vi "raster-scanning.vi"() -> ()   [LabVIEW 2017]
uses:
  controls/boolean_info.ctl
  raster-scan-params.ctl
  controls/PI-params.ctl
  <vilib>/rvi/Emulation/niFpgaGetClockAttributes.vi
  <vilib>/rvi/Emulation/niFpgaSctlEmulationGetInTimedLoop.vi
  <vilib>/rvi/Emulation/niFpgaEmulationReportErrorSimple.vi
  <vilib>/rvi/eio/common/nirviEmuTemplateMethod_errors.vi
  <vilib>/rvi/Emulation/niFpgaEmulationIsFPGAContextNoSignature.vi
  <vilib>/rvi/DataTransferAndStorage/Container/Common/niFpgaContainerGetUniqueNameForEmu.vi
  <vilib>/rvi/Memory/Memory_Emulation/niFpgaMemoryEmulationCacheClearOnFirstRun.vi
  <vilib>/rvi/Memory/Memory_Emulation/nirvimemoryEmulationManagerCache_MakeExclusive.vi
  <vilib>/rvi/Memory/Memory_Emulation/niFpgaMemoryEmulationValidateCache.vi
  <vilib>/rvi/Memory/Memory_Emulation/nirvimemoryEmulationManagerCache_InsertValue.vi
  <vilib>/Utility/error.llb/Clear Errors.vi
  <vilib>/rvi/Memory/Memory_Emulation/nirvimemoryEmulationManagerCache_ReleaseExclusive.vi
  <vilib>/rvi/Memory/Memory_Emulation/nirvimemoryEmulationManagerCache_GetValue.vi
  <vilib>/rvi/Memory/Memory_Emulation/nirvimemoryEmulationManagerCache_SetValue.vi
  <vilib>/rvi/Emulation/niFpgaProcessEmulError.vi
  <vilib>/rvi/DataTransferAndStorage/Container/Common/niFpgaContainerExecOnDevCompGetState.vi
  <vilib>/rvi/Emulation/niFpgaCriticalErrorInLSC.vi
  <vilib>/eio/EIONode/EIONode.xnode
  <vilib>/rvi/DataTransferAndStorage/Container/XNode/niFpgaContainer.xnode
  <vilib>/rvi/DataTransferAndStorage/Register/Emulation/niFpgaRegisterEmulation.vi
  <vilib>/rvi/DataTransferAndStorage/Register/Emulation/niFpgaRegisterEmulationRefIn.vi
  libimaging-cs.lvlib
  FPGA-data-logging.lvlib
panel:
  in  "ze_sched_thresh":sgl
  in  "KI_derate":sgl
  in  "raster-scan-params":T1={"TsTicks"=1600, "Stop"=TRUE, "TOL"=0.3, "ramp-rate"=0.0, "z-u-max"=5.0, "PI-params"={"Ki"=0.001, "setpoint"=0.0}, "Num"=[-0.00254, 0.000408, 0.00295, 0.0, 0.0, 0.0, 0.0, 0.0, 0.0], "TF Order"=2, "Den"=[0.982758, -1.98194, 1.0, 0.0, 0.0, 0.0, 0.0, 0.0, 0.0]} {"z-u-max" format="%#_13g"; "TOL" format="%#_13g"}
  in  "Z-settle-N":i16
  in  "do_xy_CL":bool
  in  "do-Dz":bool
  out "boolean errors":T3
  in  "xy-init":fxp<+/-,16,5>[](array[numeric])=[0.0, 0.0]
  in  "Ki-xy":sgl=0.001 format="%#_13g"
  in  "xy-bound":sgl
  in  "trigger-0":bool
  in  "u(0)":sgl format="%#_13g"
  out "e(0) (threshhold init)":fxp<+/-,16,5>
  out "current-case":i16
  out "DAC-zaxis":sgl
  out "ADC-zaxis":fxp<+/-,24,5>
  in  "raise-constant":sgl
  # "DIAGNOSTICS"
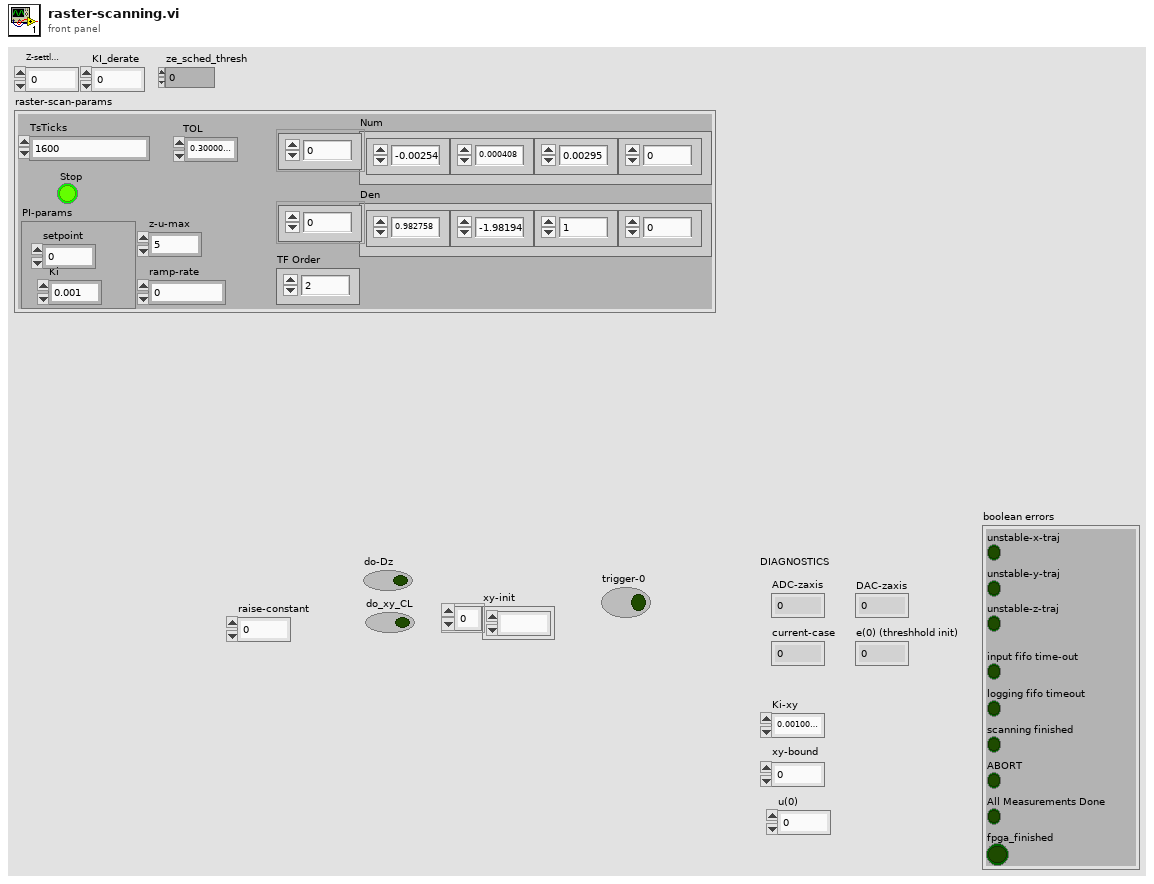
[diagram p1: front panel]
types:
  T1 = typedef "raster-scan-params.ctl" = cluster{"TsTicks":u32, "Stop":bool, "TOL":sgl, "ramp-rate":sgl, "z-u-max":sgl, "PI-params":T2, "Num":sgl[], "TF Order":i32, "Den":sgl[]}
  T2 = typedef "PI-params.ctl" = cluster{"Ki":sgl, "setpoint":sgl}
  T3 = typedef "boolean_info.ctl" = cluster{"unstable-z-traj":bool, "input fifo time-out":bool, "logging fifo timeout":bool, "scanning finished":bool, "unstable-x-traj":bool, "unstable-y-traj":bool, "ABORT":bool, "All Measurements Done":bool, "fpga_finished":bool}
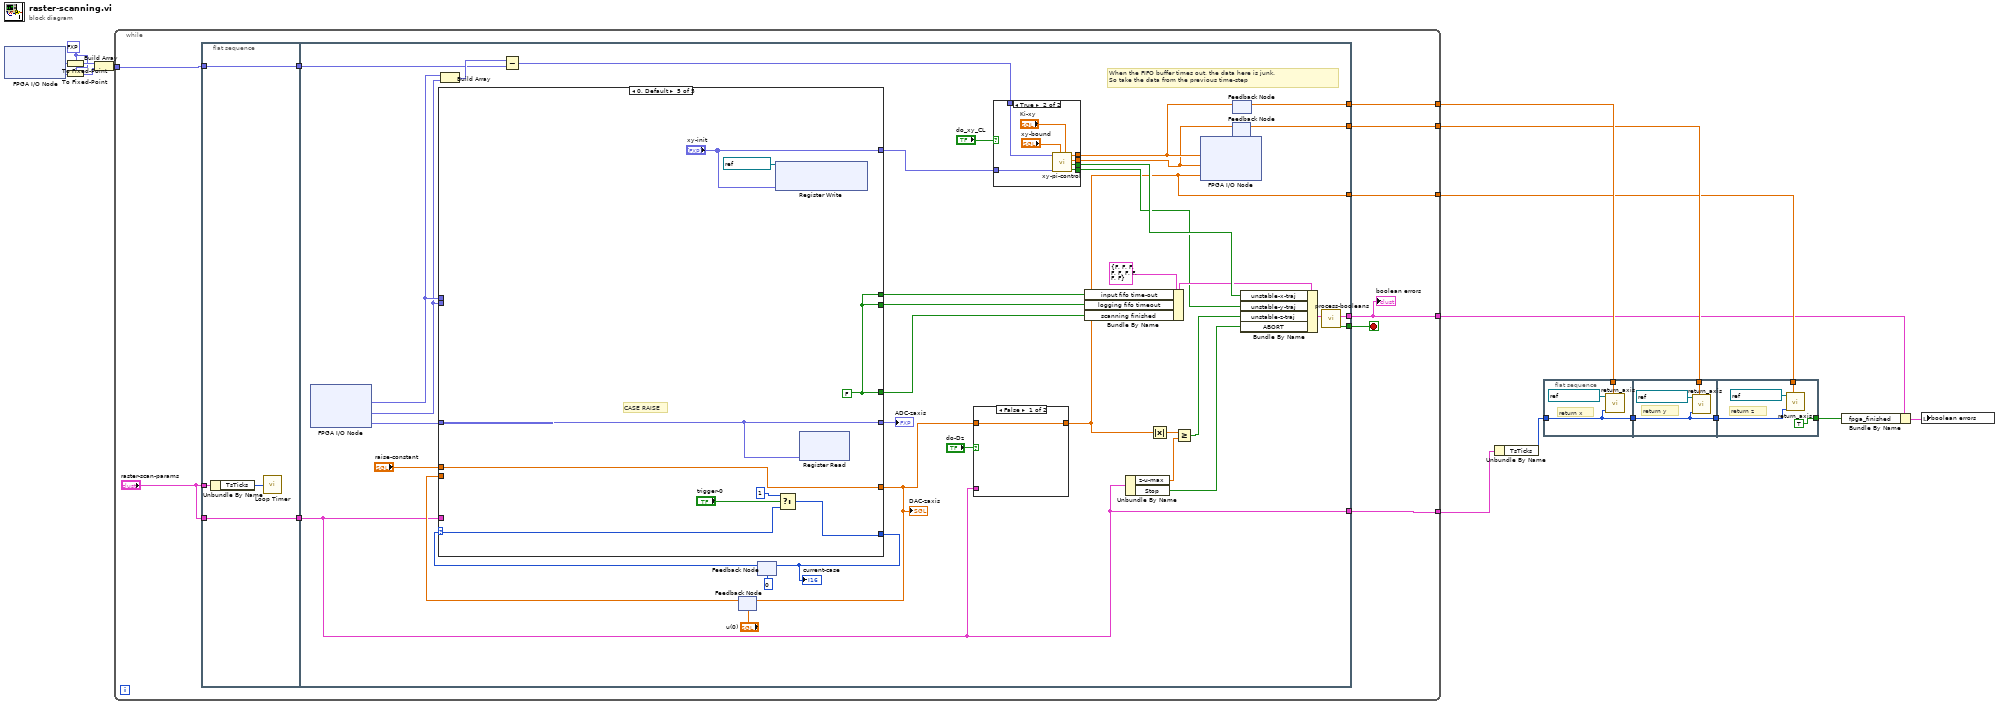
[diagram p0: block diagram]
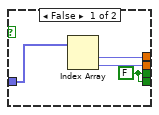
[diagram p2: hidden frame]
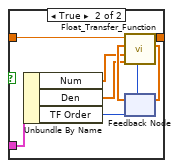
[diagram p3: hidden frame]
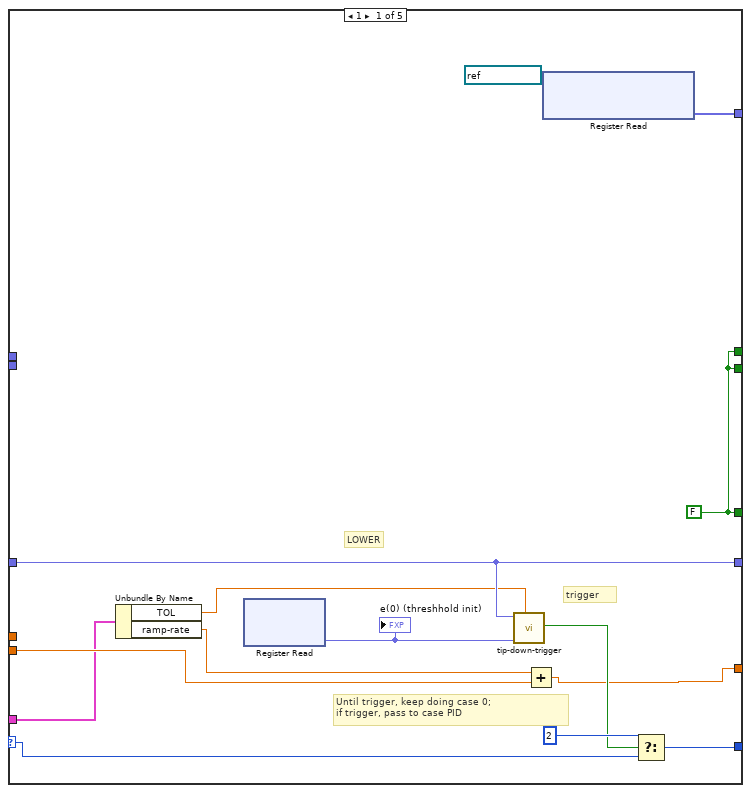
[diagram p4: hidden frame]
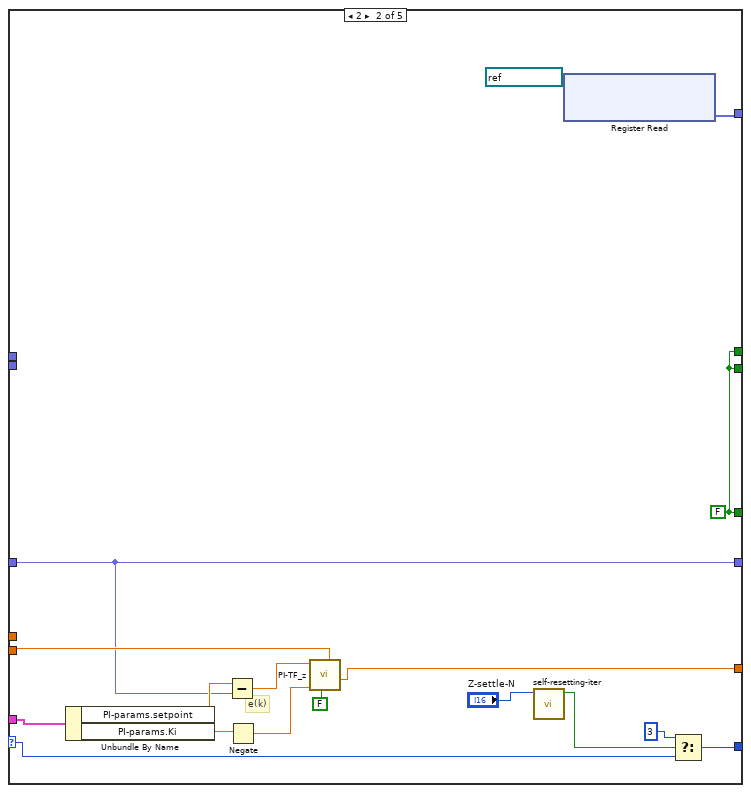
[diagram p5: hidden frame]
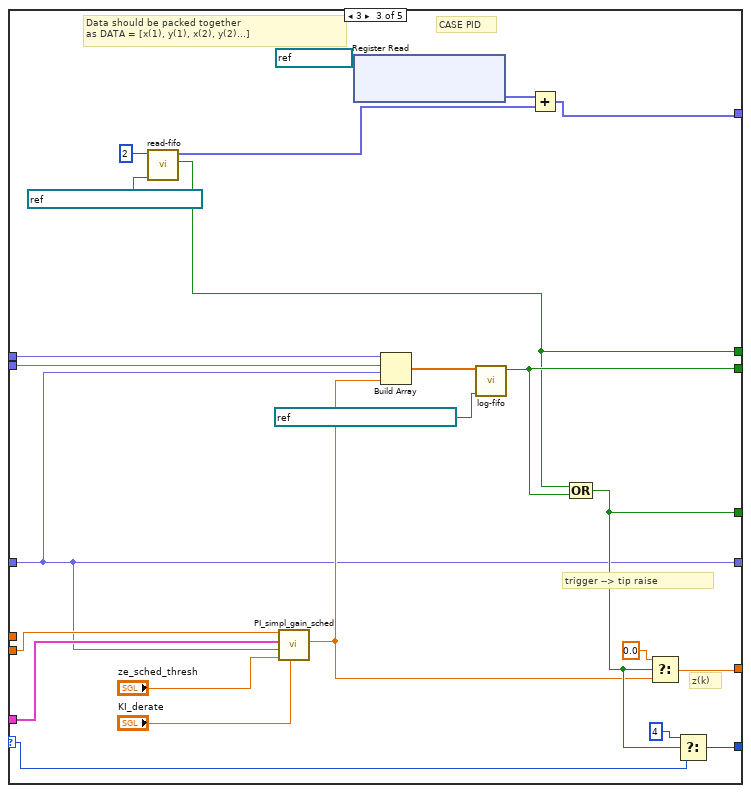
[diagram p6: hidden frame]
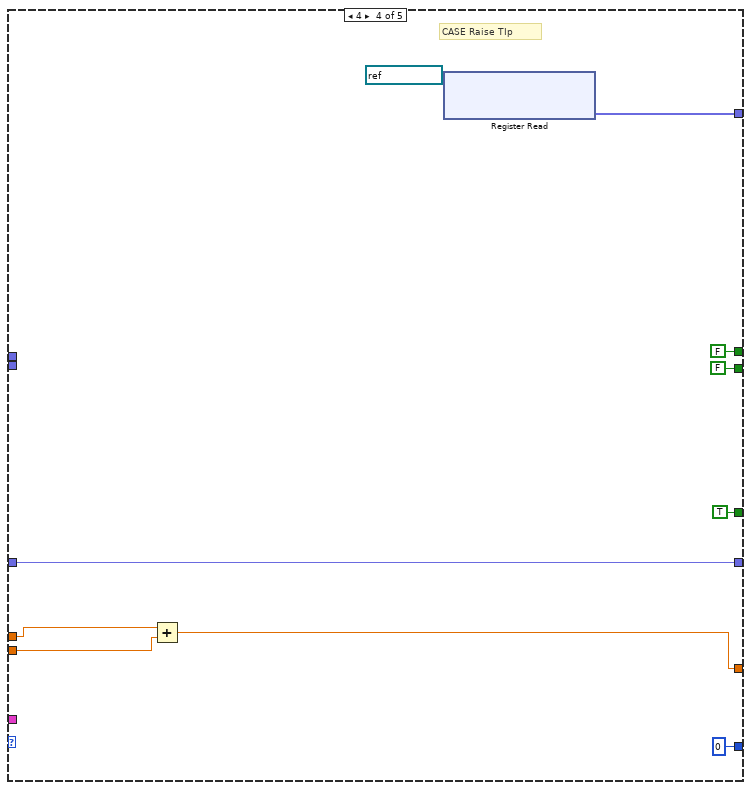
[diagram p7: hidden frame]
diagram:
  w2 = fxp<+/-,16,5> 0.0 ("fixed-point type")
  n1 = xnode "FPGA I/O Node"() -> ("Mod2/AI0"=w5:fxp<+/-,24,5>, "Mod2/AI1"=w3:fxp<+/-,24,5>)  [unwired: 2 in, 2 out]
  n2 = To Fixed-Point(fixed-point type=w2, number=w5) -> (fixed-point=w6:fxp<+/-,16,5>)
  n3 = To Fixed-Point(fixed-point type=w2, number=w3) -> (fixed-point=w4:fxp<+/-,16,5>)
  n4 = Build Array(w6, w4) -> (w1:fxp<+/-,16,5>[])
  n5 = while {
    tunnel: [w25] -> w16
    tunnel: [w24] -> w14
    tunnel: [w21] -> w8
    tunnel: [w23] -> w12
    tunnel: [w22] -> w13
    tunnel: w1 -> [w19]
    stop <- w18 stop-if-true
    n6 = flat-sequence {
      tunnel: "raster-scan-params" -> [w29]
      tunnel: [w28] -> w26
      tunnel: "raster-scan-params" -> [w28]
      tunnel: w19 -> [w27]
      tunnel: [w27] -> w20
      tunnel: w26 -> [w37]
      tunnel: [w59] -> w24
      tunnel: [w37] -> w25
      tunnel: [w33] -> w21
      tunnel: [w39] -> w23
      tunnel: [w52] -> w22
      tunnel: w20 -> [w46]
      tunnel: [w31] -> w18
      frame #0 {
        n7 = Unbundle By Name(w29) -> ("TsTicks"=w30:u32)
        n8 = call "Loop Timer"("Count(Ticks)"=w30) -> ()  [unwired: 1 out]
      }
      frame #1 {
        # "When the FIFO buffer times out, the data here is junk.\nSo take the data from the previous time-step"
        n9 = xnode "FPGA I/O Node"() -> ("Mod2/AI0"=w56:fxp<+/-,24,5>, "Mod2/AI1"=w55:fxp<+/-,24,5>, "Mod2/AI2"=w67:fxp<+/-,24,5>)  [unwired: 3 in, 3 out]
        n10 = Build Array(w56, w55) -> (w47:fxp<+/-,24,5>[])
        n11 = Subtract(x=w47, y=w46) -> (x-y=w45:fxp<+/-,25,6>[])
        n12 = feedback #1("u(0)") -> (w62:sgl)
        n13 = feedback #2(i16 0 ("f")) -> (w63:i16)
        n14 = case shown="0, Default" w63 {
          selector: w63 -> [w91 w108 w136 _ w157]
          tunnel: w62 -> [w102 w113 w124 w152 _]
          tunnel: w67 -> [w99 w106 w122 w146 w162]
          tunnel: [w99 w106 w122 w146 w162] -> w66
          tunnel: [w101 w110 w142 i16 0 ("f") w160] -> w64
          tunnel: w55 -> [_ _ w140 _ _]
          tunnel: w56 -> [_ _ w139 _ _]
          tunnel: [w92 w105 w137 TRUE ("Timed Out?") w159] -> w32
          tunnel: [w96 w112 w138 w151 w156] -> w38
          tunnel: w37 -> [w95 w114 w123 _ _]
          tunnel: [w92 w105 w130 FALSE ("Timed Out?") w159] -> w43
          tunnel: [w92 w105 w134 FALSE ("Timed Out?") w159] -> w44
          tunnel: [w89 w103 w127 w144 "xy-init"] -> w51
          tunnel: "raise-constant" -> [_ _ _ w153 w156]
          frame 1 {
            w92 = FALSE ("Timed Out?")
            # "Until trigger, keep doing case 0;\nif trigger, pass to case PID"
            # "LOWER"
            # "trigger"
            n15 = Unbundle By Name(w95) -> ("TOL"=w94:sgl, "ramp-rate"=w93:sgl)
            n16 = xnode ("Register Read")() -> ("Data"=w97:fxp<+/-,16,5>)  [unwired: 1 in, 1 out]
            "e(0) (threshhold init)" <- w97
            n17 = call "tip-down-trigger.vi"("TOL"=w94, "Vo"=w97, "e(k)"=w99) -> ("trigger"=w98:bool)  [unwired: 8 in]
            n18 = Add(x=w93, y=w102) -> (x+y=w96:sgl)
            n19 = xnode ("Register Read")("Register In"=refnum<k21> "xy_init") -> ("Data"=w89:fxp<+/-,17,6>[])  [unwired: 1 out]
            n20 = Select(t=i16 2, s=w98, f=w91) -> (s? t:f=w101:i16)
          }
          frame 2 {
            w105 = FALSE ("Timed Out?")
            # "e(k)"
            n21 = Unbundle By Name(w114) -> ("PI-params.setpoint"=w119:sgl, "PI-params.Ki"=w116:sgl)
            n22 = Subtract(x=w119, y=w106) -> (x-y=w117:sgl)
            n23 = Negate(x=w116) -> (-x=w115:sgl)
            n24 = call "PI-TF_z.vi"("u(k-1)"=w113, "reset"=FALSE, "Ki"=w115, "e(k)"=w117) -> ("u(k)"=w112:sgl)  [unwired: 7 in]
            n25 = call "self-resetting-iter.vi"("N"="Z-settle-N") -> ("Boolean"=w109:bool)  [unwired: 9 in, 1 out]
            n26 = xnode ("Register Read")("Register In"=refnum<k21> "xy_init") -> ("Data"=w103:fxp<+/-,17,6>[])  [unwired: 1 out]
            n27 = Select(t=i16 3, s=w109, f=w108) -> (s? t:f=w110:i16)
          }
          frame 3 {
            # "Data should be packed together\nas DATA = [x(1), y(1), x(2), y(2)...]"
            # "trigger --> tip raise"
            # "z(k)"
            # "CASE PID"
            n28 = call "read-fifo.vi"("FIFO In"=refnum<k21> "host-to-fpga-fxp-16-5", "numChan"=2) -> ("timout?"=w130:bool, "unpacked-data"=w126:fxp<+/-,16,5>[])  [unwired: 8 in]
            n29 = call "PI_simpl_gain_sched.vi"("KI_derate"="KI_derate", "ze_sched_thresh"="ze_sched_thresh", "ze"=w122, "raster-scan-params"=w123, "u(k-1)"=w124) -> ("u(k)"=w125:sgl)  [unwired: 6 in]
            n30 = xnode ("Register Read")("Register In"=refnum<k21> "xy_init") -> ("Data"=w128:fxp<+/-,17,6>[])  [unwired: 1 out]
            n31 = Build Array(w139, w140, w122, w125) -> (w135:sgl[])
            n32 = call "log-fifo.vi"("FIFO In"=refnum<k21> "fpga-to-host2-fxp-16-5", "input-data"=w135) -> ("logging-timeout?"=w134:bool)  [unwired: 9 in]
            n33 = Add(x=w128, y=w126) -> (x+y=w127:fxp<+/-,18,7>[])
            n34 = Compound Arithmetic op=OR(w130, w134) -> (w137:bool)
            n35 = Select(t=sgl 0.0 ("f"), s=w137, f=w125) -> (s? t:f=w138:sgl)
            n36 = Select(t=i16 4, s=w137, f=w136) -> (s? t:f=w142:i16)
          }
          frame 4 {
            # "CASE Raise TIp"
            n37 = Add(x=w153, y=w152) -> (x+y=w151:sgl)
            n38 = xnode ("Register Read")("Register In"=refnum<k21> "xy_init") -> ("Data"=w144:fxp<+/-,17,6>[])  [unwired: 1 out]
          }
          frame 0, Default {
            w159 = FALSE ("Timed Out?")
            # "CASE RAISE"
            n39 = xnode ("Register Write")("Data"="xy-init", "Register In"=refnum<k21> "xy_init") -> ()  [unwired: 1 out]
            n40 = Select(t=i16 1 ("f"), s="trigger-0", f=w157) -> (s? t:f=w160:i16)
            n41 = xnode ("Register Read")("Data"=w162) -> ()  [unwired: 1 in, 1 out]
          }
        }
        "ADC-zaxis" <- w66
        "DAC-zaxis" <- w38
        "current-case" <- w64
        n42 = feedback-in #1(w38) -> ()
        n43 = feedback-in #2(w64) -> ()
        n44 = case shown="False" "do-Dz" {
          tunnel: [w80 w86] -> w39
          tunnel: w38 -> [w80 w85]
          tunnel: w37 -> [_ w81]
          frame False {
          }
          frame True {
            n45 = Unbundle By Name(w81) -> ("Num"=w84:sgl[], "Den"=w83:sgl[], "TF Order"=w82:i32)
            n46 = feedback #3() -> (w87:sgl[])  [unwired: 1 in]
            n47 = call "Float_Transfer_Function.vi"("TF Order"=w82, "Den"=w83, "Num"=w84, "State In"=w87, "Input"=w85) -> ("State Out"=w88:sgl[], "Output"=w86:sgl)  [unwired: 4 in]
            n48 = feedback-in #3(w88) -> ()
          }
        }
        n49 = case shown="True" "do_xy_CL" {
          tunnel: [w70 w77] -> w54
          tunnel: [w69 w76] -> w53
          tunnel: w51 -> [w71 w75]
          tunnel: [w68 w74] -> w49
          tunnel: w45 -> [_ w73]
          tunnel: [w68 w72] -> w40
          frame False {
            w68 = FALSE ("u_x saturated")
            n50 = Index Array(array=w71) -> (element #1=w70:fxp<+/-,18,7>, element #2=w69:fxp<+/-,18,7>)  [unwired: 2 in]
          }
          frame True {
            n51 = call "xy-pi-control.vi"("Ki-xy"="Ki-xy", "xy-umax"="xy-bound", "xy-ref"=w75, "x_k-y_k"=w73) -> ("u_y saturated"=w72:bool, "u_x saturated"=w74:bool, "sat(u_y)"=w76:sgl, "sat(u_x)"=w77:sgl)  [unwired: 4 in]
          }
        }
        n52 = Bundle By Name(cluster=T3 {"unstable-z-traj"=FALSE, "input fifo time-out"=FALSE, "logging fifo timeout"=FALSE, "scanning finished"=FALSE, "unstable-x-traj"=FALSE, "unstable-y-traj"=FALSE, "ABORT"=FALSE, "All Measurements Done"=FALSE, "fpga_finished"=FALSE} ("boolean errors 2"), "input fifo time-out"=w43, "logging fifo timeout"=w44, "scanning finished"=w32) -> (w41:T3)
        n53 = Unbundle By Name(w37) -> ("z-u-max"=w60:sgl, "Stop"=w57:bool)
        n54 = Absolute Value(x=w39) -> (abs(x)=w65:sgl)
        n55 = Greater Or Equal?(x=w65, y=w60) -> (x >= y?=w58:bool)
        n56 = xnode "FPGA I/O Node"("Mod1/AO0"=w54, "Mod1/AO1"=w53, "Mod1/AO2"=w39) -> ()  [unwired: 3 in, 3 out]
        n57 = feedback #4() -> (w52:sgl)  [unwired: 1 in]
        n58 = feedback-in #4(w53) -> ()
        n59 = feedback-in #5(w54) -> ()
        n60 = feedback #5() -> (w59:sgl)  [unwired: 1 in]
        n61 = Bundle By Name(cluster=w41, "unstable-x-traj"=w49, "unstable-y-traj"=w40, "unstable-z-traj"=w58, "ABORT"=w57) -> (w34:T3)
        n62 = call "process-booleans.vi"("boolean indicators 2"=w34) -> ("scaning finished"=w31:bool, "boolean indicators"=w33:T3)  [unwired: 9 in]
      }
    }
    "boolean errors" <- w21
  }
  n63 = Unbundle By Name(w16) -> ("TsTicks"=w15:u32)
  n64 = flat-sequence {
    tunnel: w15 -> [w164]
    tunnel: w14 -> [w165]
    tunnel: [w164] -> w11
    tunnel: w13 -> [w168]
    tunnel: w11 -> [w166]
    tunnel: [w166] -> w10
    tunnel: w12 -> [w172]
    tunnel: w10 -> [w170]
    tunnel: [TRUE] -> w9
    frame #0 {
      # "return x"
      n65 = call "return_axis.vi"("u(0)"=w165, "TsTicks"=w164, "FPGA I/O In"=refnum<k21> "Mod1/AO0") -> ()  [unwired: 9 in]
    }
    frame #1 {
      # "return y"
      n66 = call "return_axis.vi"("u(0)"=w168, "TsTicks"=w166, "FPGA I/O In"=refnum<k21> "Mod1/AO1") -> ()  [unwired: 9 in]
    }
    frame #2 {
      # "return z"
      n67 = call "return_axis.vi"("u(0)"=w172, "TsTicks"=w170, "FPGA I/O In"=refnum<k21> "Mod1/AO2") -> ()  [unwired: 9 in]
    }
  }
  n68 = Bundle By Name(cluster=w8, "fpga_finished"=w9) -> (w7:T3)
  n69 = local write "boolean errors"(w7) -> ()
